vi "Read outputs.vi"(8 "error in":errorcluster, 11 "shared memory module runtime":refnum<class "Shared Memory Runtime.lvclass">) -> (0 "error out":errorcluster, 2 "outputs":T1[](array[typedef]), 3 "shared memory module runtime out":refnum<class "Shared Memory Runtime.lvclass">)   [LabVIEW 2013, in "Shared Memory Runtime.lvclass"]
uses:
  Shared Memory Runtime.lvclass
  shared memory module runtime.ctl
  <vilib>/NI/Tag Bus Module Framework/channel/channel classification.ctl
  <vilib>/NI/Tag Bus/tag/Data Type.ctl
  <vilib>/National Instruments/Shared Memory Library for Linux RT/Controls/Shared Memory Data.ctl
  Shared Memory Runtime.lvclass/Shared Memory Runtime.ctl
  <vilib>/NI/Tag Bus/tag/tag descriptor.lvclass
  <vilib>/National Instruments/Shared Memory Library for Linux RT/Shared Memory.lvlib
  <vilib>/NI/Tag Bus Module Framework/channel/TBM channel.lvclass
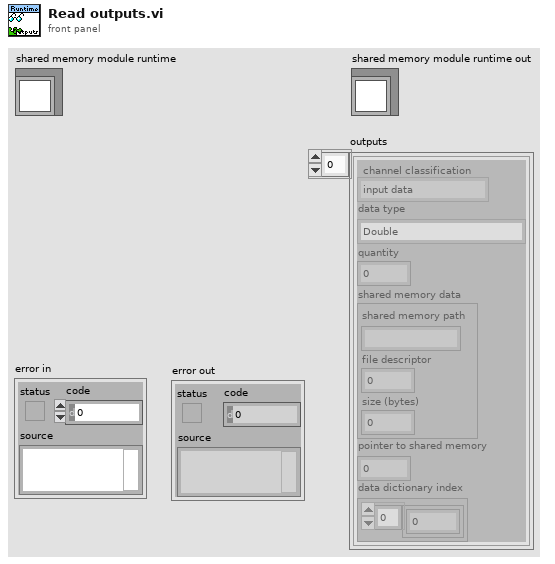
[diagram p1: front panel]
types:
  T1 = typedef "Shared Memory Runtime.lvclass/shared memory module runtime.ctl" = cluster{"channel classification":T2, "data type":T3, "quantity":u16, "shared memory data":T4, "pointer to shared memory":u64, "data dictionary index":cluster{i32[]}}
  T2 = typedef "TBM channel.lvclass/channel classification.ctl" = enum16{"input data", "output data", "processing parameter", "processing result"}
  T3 = typedef "tag bus.lvlib/tag descriptor.lvclass/Data Type.ctl" = enum16{"Double", "Single", "I64", "I32", "I16", "I8", "U64", "U32", "U16", "U8", "Boolean", "String", "Array of Double", "Array of Single", "Array of I64", "Array of I32", "Array of I16", "Array of I8", "Array of U64", "Array of U32", "Array of U16", "Array of U8", "Array of Boolean", "Array of String"}
  T4 = typedef "Shared Memory.lvlib/Shared Memory Data.ctl" = cluster{"shared memory path":string, "file descriptor":i32, "size (bytes)":u32}
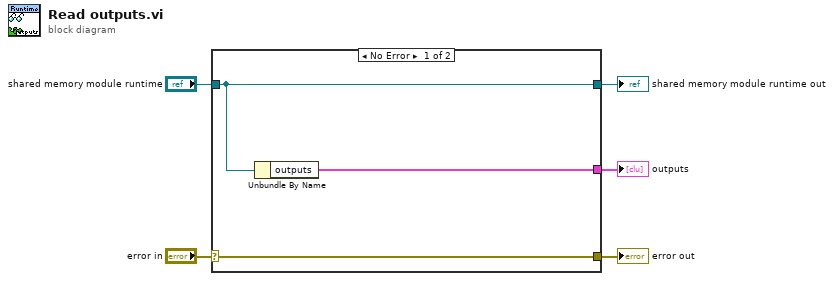
[diagram p0: block diagram]
diagram:
  n1 = case shown="No Error" "error in" {
    selector: "error in" -> [w8 w9]
    tunnel: [w8 w9] -> w4
    tunnel: [w7 w10] -> w2
    tunnel: "shared memory module runtime" -> [w7 w10]
    tunnel: [w6 _] -> w1
    frame No Error {
      n2 = Unbundle By Name(w7) -> ("outputs"=w6:T1[])
    }
    frame Error {
    }
  }
  "error out" <- w4
  "shared memory module runtime out" <- w2
  "outputs" <- w1
